vi "Autonomous Independent.vi"() -> ()   [LabVIEW 2013]
doc: "This VI is called when autonomous begins, and will automatically be terminated when autonomous ends. You can carry out timed or sensor driven robot movement independently without needing to return to the caller."
uses:
  Robot Global Data.vi
  AutoState.ctl
  DoubleSolenoidControl.ctl
  Roller States.ctl
panel:
  out "Error out":errorcluster
  in  "Error in":errorcluster
  # "Be sure to right-click and choose Data Operations>>Make Current Value default if you want to save the array values with the VI"
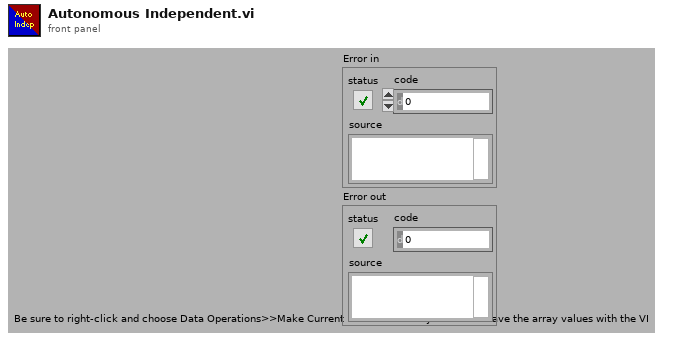
[diagram p1: front panel]
types:
  T1 = typedef "AutoState.ctl" = enum16{"One Ball", "Two Ball"}
  T2 = typedef "WPI_JoystickDevRef.ctl" = cluster{"Device":T3}
  T3 = typedef "WPI_JoystickDeviceEnum.ctl" = enum16{"USB 1", "USB 2", "USB 3", "USB 4", "Kinect 1", "Kinect 2"}
  T4 = cluster{"axis 1 (x)":dbl, "axis 2 (y)":dbl, "axis 3 (throttle)":dbl, "axis 4":dbl, "axis 5":dbl, "axis 6":dbl}
  T5 = typedef "DoubleSolenoidControl.ctl" = enum16{"Init", "Out", "In", "Middle"}
  T6 = typedef "Roller States.ctl" = enum16{"Off", "Forward", "Reverse"}
  T7 = typedef "WPI_RelayDevRef.ctl" = cluster{"DevStatus":errorcluster, "Relay Channel":T8, "Digital Module":T9, "Relay Direction":T10}
  T8 = typedef "FPGA_DIORelayChannel.ctl" = enum8{"Relay 1", "Relay 2", "Relay 3", "Relay 4", "Relay 5", "Relay 6", "Relay 7", "Relay 8", "Invalid"}
  T9 = typedef "FPGA_TypedefDigitalModule.ctl" = enum16{"Digital Module 1", "Digital Module 2"}
  T10 = typedef "WPI_RelayDirection.ctl" = enum16{"Both directions", "Forward only", "Reverse only"}
  T11 = typedef "WPI_SolenoidDevRef.ctl" = cluster{"DevStatus":errorcluster, "Solenoid Module":T12, "Forward Solenoid Channel":T13, "Reverse Solenoid Channel":T13}
  T12 = typedef "FPGA_TypedefSolenoidModule.ctl" = enum16{"Solenoid Module 1", "Solenoid Module 2"}
  T13 = typedef "WPI_SolenoidChannel.ctl" = enum8{"Solenoid 1", "Solenoid 2", "Solenoid 3", "Solenoid 4", "Solenoid 5", "Solenoid 6", "Solenoid 7", "Solenoid 8", "Invalid"}
  T14 = typedef "WPI_MotorControlDeviceRef.ctl" = cluster{"DeviceStatus":errorcluster, "Type":enum16{"PWM", "CAN"}, "PWM":cluster{"Digital Module":T9, "PWM Channel":T15, "DeadBand":T16}, "CAN":cluster{"Device Number":u8, "Control Mode":T17, "Semaphore":T18, "Max Vout":dbl}, "Invert":bool, "TransformRef":T19, "InvTransformRef":T19}
  T15 = typedef "FPGA_DIOPWMChannel.ctl" = enum8{"PWM 1", "PWM 2", "PWM 3", "PWM 4", "PWM 5", "PWM 6", "PWM 7", "PWM 8", "PWM 9", "PWM 10", "Invalid"}
  T16 = typedef "WPI_PWMDeadband.ctl" = cluster{"Name":string, "maxPositivePwm":i32, "minPositivePwm":i32, "centerPwm":i32, "maxNegativePwm":i32, "minNegativePwm":i32, "angularRange":u16}
  T17 = typedef "WPI_CANJaguar_ControlMode.ctl" = enum8{"Percent VBus", "Current", "Speed", "Position", "Voltage"}
  T18 = typedef "Semaphore RefNum" = refnum<k1>
  T19 = typedef "WPI_PWMTransform_ConPane.ctl" = refnum<vi>
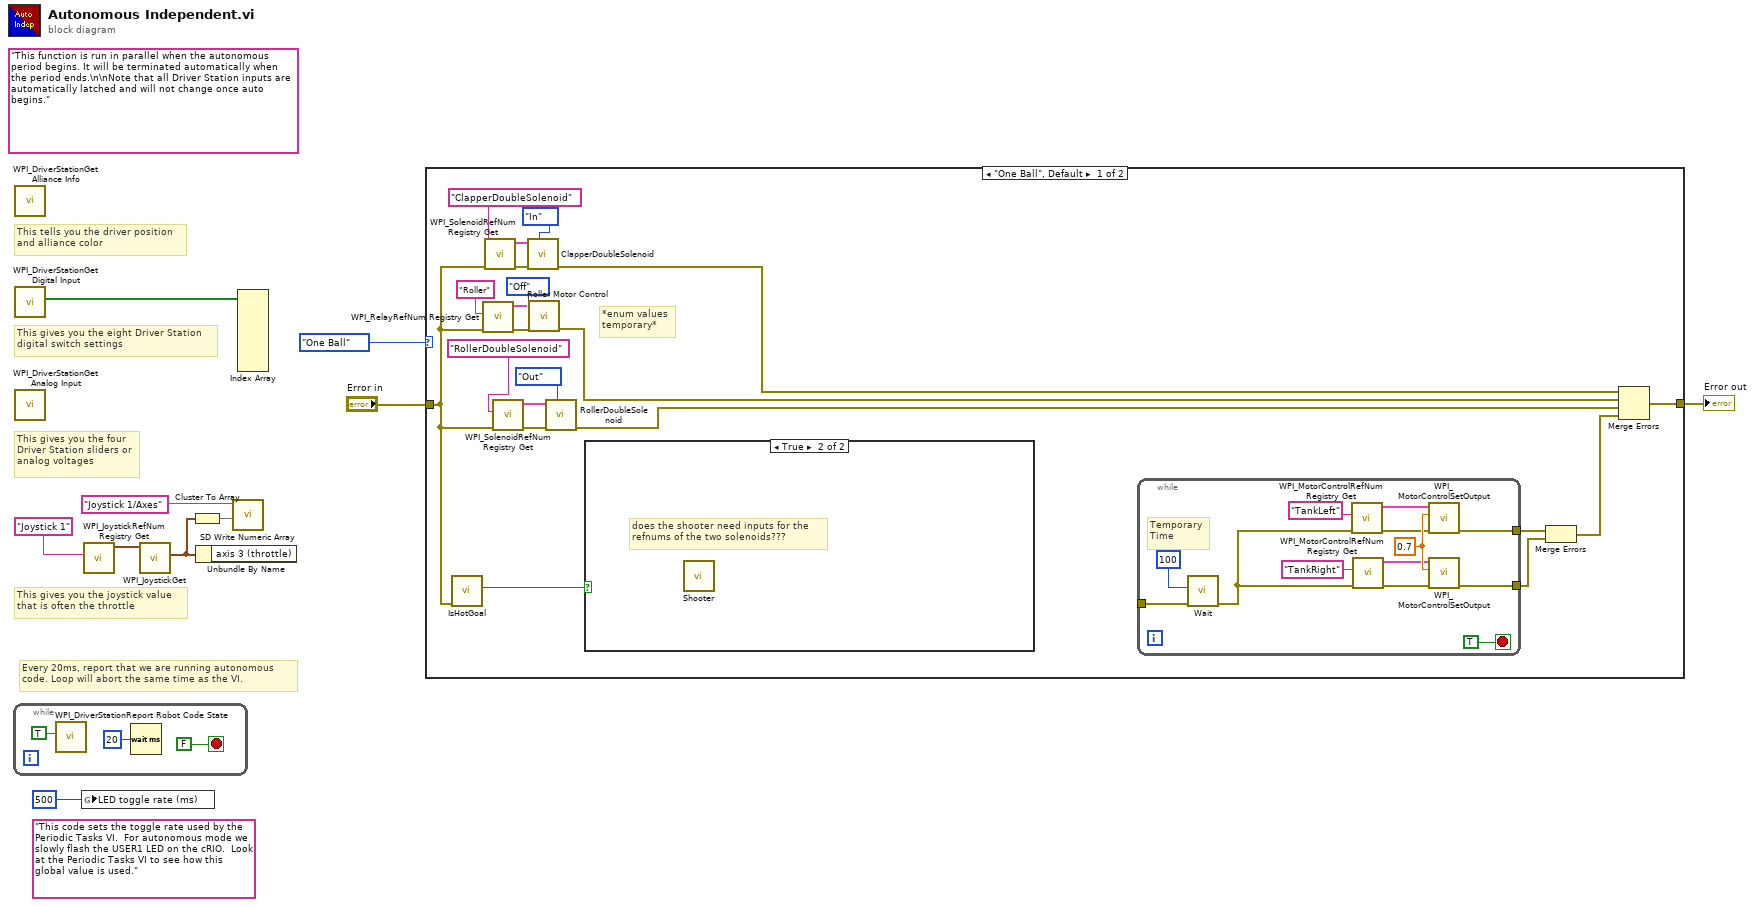
[diagram p0: block diagram]
diagram:
  (unwired) "This code sets the toggle rate used by the Periodic Tasks VI.  For autonomous mode we slowly flash the USER1 LED on the cRIO.  Look at the Periodic Tasks VI to see how this global value is used."
  (unwired) "This function is run in parallel when the autonomous period begins. It will be terminated automatically when the period ends.\n\nNote that all Driver Station inputs are automatically latched and will not change once auto begins."
  # "Every 20ms, report that we are running autonomous\ncode. Loop will abort the same time as the VI."
  # "This gives you the joystick value\nthat is often the throttle"
  # "This tells you the driver position\nand alliance color"
  # "This gives you the eight Driver Station\ndigital switch settings"
  # "This gives you the four\nDriver Station sliders or\nanalog voltages"
  n1 = while {
    stop <- FALSE stop-if-true
    n2 = call <vilib>:"WPI_DriverStationReport Robot Code State.vi"("Autonomous"=TRUE) -> ()  [unwired: 10 in, 1 out]
    n3 = Wait (ms)(milliseconds to wait=u32 20) -> ()  [unwired: 1 out]
  }
  n4 = call <vilib>:"WPI_DriverStationGet Alliance Info.vi"() -> ()  [unwired: 12 out]
  n5 = call <vilib>:"WPI_DriverStationGet Digital Input.vi"() -> ("Driver Station Digital Input (1-8)"=w10:bool[])  [unwired: 11 out]
  n6 = call <vilib>:"WPI_DriverStationGet Analog Input.vi"() -> ()  [unwired: 12 out]
  n7 = global write "Robot Global Data.vi" "LED toggle rate (ms)"(u32 500 ("LED ms toggle rate")) -> ()
  n8 = call <vilib>:"WPI_JoystickRefNum Registry Get.vi"("refnum name"="Joystick 1") -> ("JoystickDevRef"=w8:T2)  [unwired: 1 in, 9 out]
  n9 = call <vilib>:"WPI_JoystickGet.vi"("JoystickDevRef"=w8) -> ("Axes"=w5:T4)  [unwired: 1 in, 5 out]
  n10 = Cluster To Array(cluster=w5) -> (array=w6:dbl[])
  n11 = Unbundle By Name(w5) -> ()  [unwired: 1 out]
  n12 = call <vilib>:"SD Write Numeric Array.vi"("Numeric Array"=w6, "Name"="Joystick 1/Axes") -> ()  [unwired: 8 in, 2 out]
  n13 = Index Array(array=w10) -> ()  [unwired: 8 in, 8 out]
  n14 = case shown="\"One Ball\", Default" AutoState."One Ball" {
    tunnel: [w30 _] -> w2
    tunnel: "Error in" -> [w18 _]
    frame "One Ball", Default {
      # "*enum values\ntemporary*"
      n15 = call "IsHotGoal.vi"("error in"=w18) -> ("Hot/Not"=w14:bool)  [unwired: 9 in, 1 out]
      n16 = call <vilib>:"WPI_RelayRefNum Registry Get.vi"("error in (no error)"=w18, "refnum name"="Roller") -> ("error out"=w27:errorcluster, "RelayDevRef"=w31:T7)  [unwired: 8 in]
      n17 = call <vilib>:"WPI_SolenoidRefNum Registry Get.vi"("error in (no error)"=w18, "refnum name"="ClapperDoubleSolenoid") -> ("error out"=w26:errorcluster, "SolenoidDevRef"=w33:T11)  [unwired: 8 in]
      n18 = call <vilib>:"WPI_SolenoidRefNum Registry Get.vi"("error in (no error)"=w18, "refnum name"="RollerDoubleSolenoid") -> ("error out"=w21:errorcluster, "SolenoidDevRef"=w22:T11)  [unwired: 8 in]
      n19 = call "ClapperDoubleSolenoid.vi"("State"=DoubleSolenoidControl."In", "Error in"=w26, "SolenoidDevRef"=w33) -> ("Error out"=w29:errorcluster)  [unwired: 8 in]
      n20 = call "Roller Motor Control.vi"("Error in"=w27, "RollerState"=Roller_States."Off", "RelayDevRef"=w31) -> ("Error out"=w28:errorcluster)  [unwired: 8 in]
      n21 = call "RollerDoubleSolenoid.vi"("State"=DoubleSolenoidControl."Out", "Error in"=w21, "SolenoidDevRef"=w22) -> ("Error out"=w20:errorcluster)  [unwired: 8 in]
      n22 = case shown="True" w14 {
        frame False {
        }
        frame True {
          # "does the shooter need inputs for the \nrefnums of the two solenoids???"
          n23 = call "Shooter.vi"() -> ()  [unwired: 11 in, 1 out]
        }
      }
      n24 = while {
        tunnel: [w39] -> w17
        tunnel: [w38] -> w16
        tunnel: _ -> [w37]
        stop <- TRUE stop-if-true
        w44 = 0.7 ("Output")
        # "Temporary\nTime"
        n25 = call "Wait.vi"("error in"=w37, "milliseconds to wait"=u32 100) -> ("error out"=w36:errorcluster)  [unwired: 9 in]
        n26 = call <vilib>:"WPI_MotorControlRefNum Registry Get.vi"("error in (no error)"=w36, "refnum name"="TankLeft") -> ("error out"=w41:errorcluster, "MotorControlDevRef"=w43:T14)  [unwired: 8 in]
        n27 = call <vilib>:"WPI_MotorControlRefNum Registry Get.vi"("error in (no error)"=w36, "refnum name"="TankRight") -> ("error out"=w40:errorcluster, "MotorControlDevRef"=w42:T14)  [unwired: 8 in]
        n28 = call <vilib>:"WPI_MotorControlSetOutput.vi"("error in (no error)"=w41, "Output"=w44, "MotorControlDevRef"=w43) -> ("error out"=w39:errorcluster)  [unwired: 6 in, 2 out]
        n29 = call <vilib>:"WPI_MotorControlSetOutput.vi"("error in (no error)"=w40, "Output"=w44, "MotorControlDevRef"=w42) -> ("error out"=w38:errorcluster)  [unwired: 6 in, 2 out]
      }
      n30 = Merge Errors(w17, w16) -> (w15:errorcluster)
      n31 = Merge Errors(w29, w28, w20, w15) -> (w30:errorcluster)
    }
    frame "Two Ball" {
    }
  }
  "Error out" <- w2
